vi "Kpro Read String Pot 2016.vi"(0 "Read String Pot":bool, 1 "Feet of\nStainless to be\nUsed (Count) in":i32, 2 "Corrected Array in":dbl[][](array[numeric]), 3 "Flow":dbl, 4 "Increment":bool, 5 "Finished In":bool, 6 "Depth Cluster in":T1, 7 "error in (no error)":errorcluster, 8 "String Pot \nSlope in":dbl=1.7339999675750732 format="%.2f", 9 "Sensor Cluster In in":T3, 10 "Descriptions":string[](array[string]), 11 "Zeroed Pressure in":dbl format="%.2f", 12 "Array in":refnum<k24>[](array[refnum]), 14 "Output KPRO in":path=path "c:/junk.dat") -> (18 "Sensor Cluster 2":T3, 19 "IK":dbl, 20 "Array out":refnum<k24>[](array[refnum]), 21 "Boolean":bool, 22 "Boolean 2":bool, 23 "Enum":T2(ring), 24 "Feet of\nStainless to be\nUsed (Count) out":i32, 25 "Depth Cluster out":T1, 26 "Corrected Array out":dbl[][](array[numeric]))   [LabVIEW 2016]
uses:
  Waterloo DAQ/controls/MCC DAQ Readings.ctl
  C:/Program Files (x86)/National Instruments/LabVIEW 2016/vi.lib/ULx/ULx_LV.dll
  Waterloo DAQ/controls/Kpro hydraulic measurement cluster.ctl
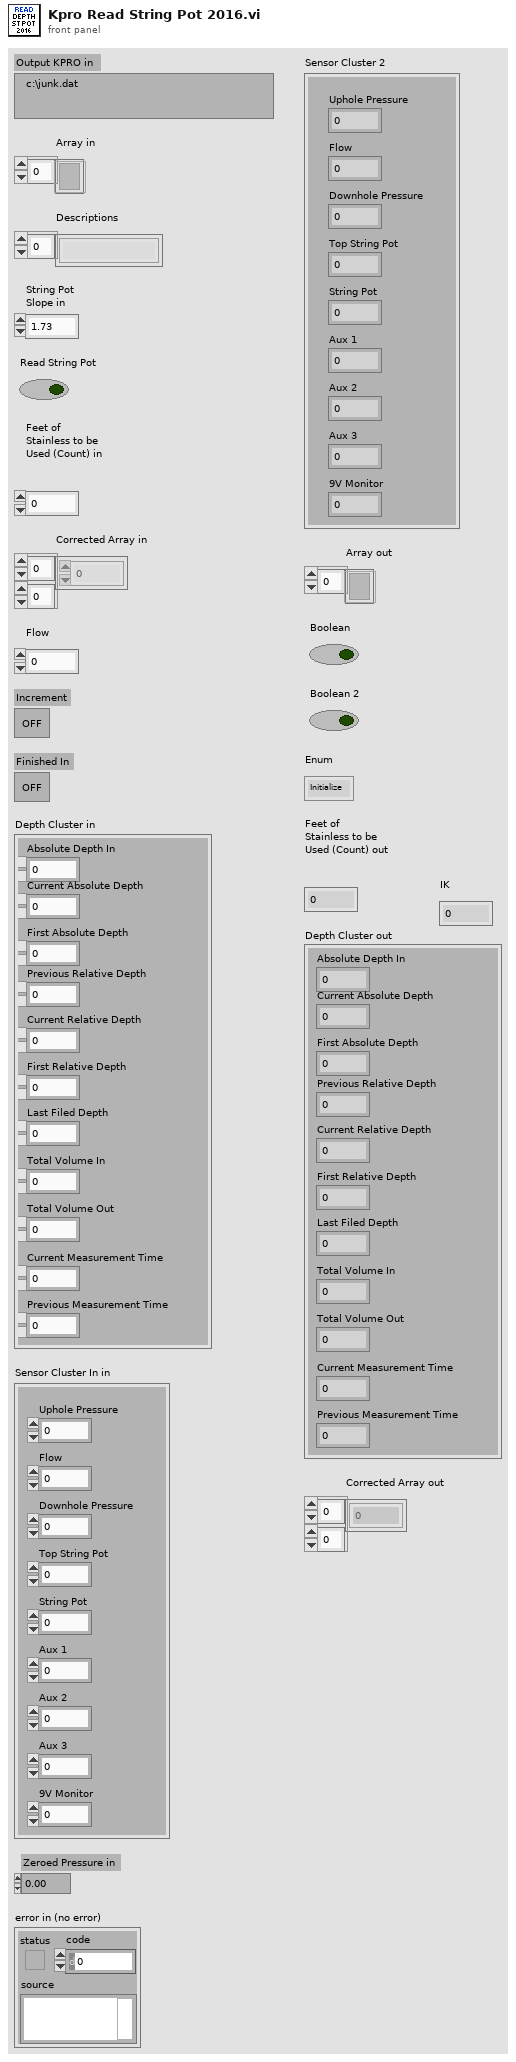
[diagram p1: front panel]
types:
  T1 = typedef "Kpro hydraulic measurement cluster.ctl" = cluster{"Absolute Depth In":dbl, "Current Absolute Depth":dbl, "First Absolute Depth":dbl, "Previous Relative Depth":dbl, "Current Relative Depth":dbl, "First Relative Depth":dbl, "Last Filed Depth":dbl, "Total Volume In":dbl, "Total Volume Out":dbl, "Current Measurement Time":dbl, "Previous Measurement Time":dbl}
  T2 = enum16{"Initialize", "Read", "Calc IK and generate Array", "Write Data & finish"}
  T3 = typedef "MCC DAQ Readings.ctl" = cluster{"Uphole Pressure":dbl, "Flow":dbl, "Downhole Pressure":dbl, "Top String Pot":dbl, "String Pot":dbl, "Aux 1":dbl, "Aux 2":dbl, "Aux 3":dbl, "9V Monitor":dbl}
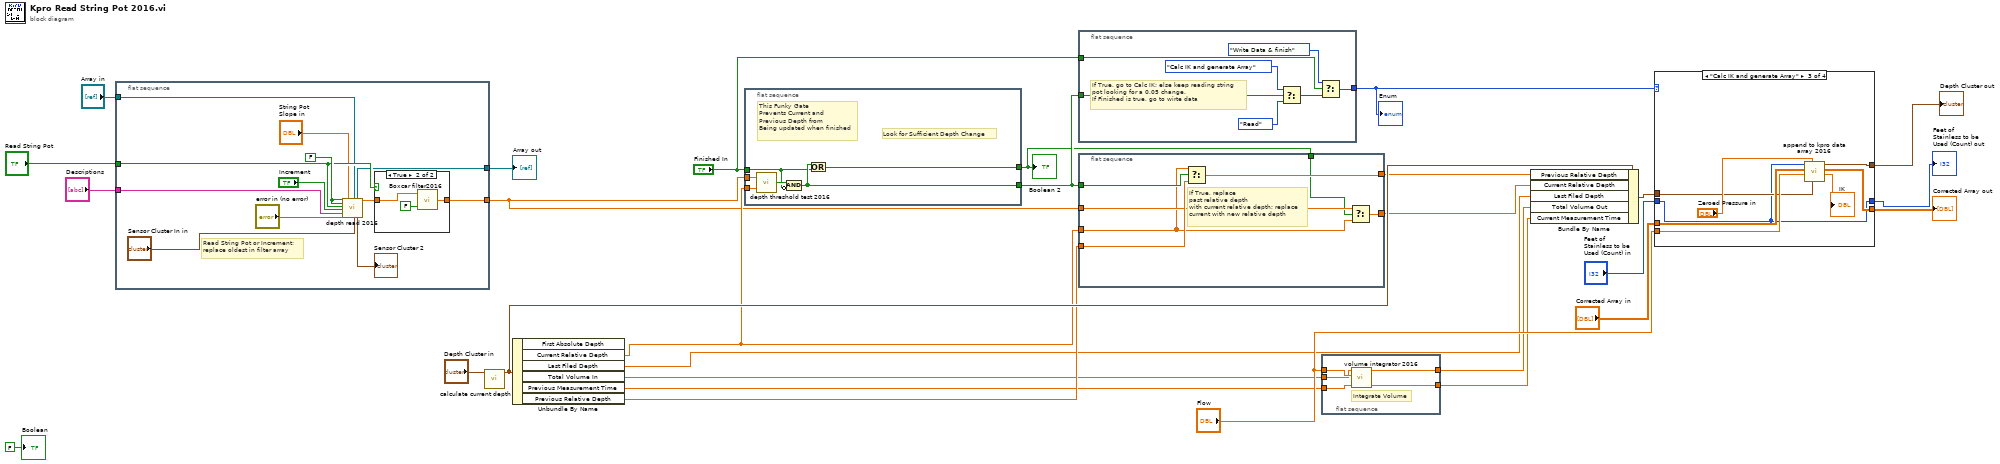
[diagram p0: block diagram]
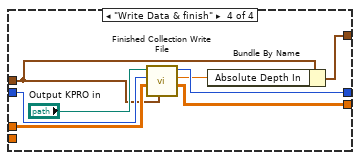
[diagram p4: hidden frame]
diagram:
  n1 = flat-sequence {
    tunnel: [w37] -> w5
    tunnel: "Read String Pot" -> [w36]
    tunnel: "Descriptions" -> [w35]
    tunnel: [w32] -> w27
    tunnel: "Array in" -> [w31]
    frame #0 {
      w39 = FALSE
      # "Read String Pot or Increment;\nreplace oldest in filter array"
      n2 = call "depth read 2016.vi"("Debug"=w39, "Initialize Debug"=w39, "Read String Pot"=w36, "Increment Button"="Increment", "Descriptions"=w35, "error in (no error)"="error in (no error)", "String Pot \nSlope"="String Pot \nSlope in", "Array in"=w31, "Sensor Cluster In"="Sensor Cluster In in") -> ("Array out"=w32:refnum<k24>[], "Sensor Cluster 2"=→"Sensor Cluster 2":T3, "Depth"=w40:dbl)  [unwired: 7 in, 1 out]
      n3 = case shown="True" w36 {
        tunnel: w40 -> [w41 w43]
        tunnel: [w41 w42] -> w37
        frame False {
        }
        frame True {
          n4 = call "Boxcar filter2016.vi"("Initialize"=FALSE, "Filter Input"=w43) -> ("Filter Output"=w42:dbl)  [unwired: 1 in]
        }
      }
    }
  }
  n5 = call "calculate current depth.vi"("Cluster in"="Depth Cluster in") -> ("Cluster out"=w17:T1)  [unwired: 10 in]
  n6 = Unbundle By Name(w17) -> ("Current Relative Depth"=w7:dbl, "Last Filed Depth"=w12:dbl, "Total Volume In"=w8:dbl, "Previous Measurement Time"=w14:dbl, "Previous Relative Depth"=w15:dbl)  [unwired: 1 out]
  n7 = flat-sequence {
    tunnel: [w49] -> w1
    tunnel: [w48] -> w2
    tunnel: "Finished In" -> [w47]
    tunnel: w5 -> [w46]
    tunnel: w7 -> [w45]
    frame #0 {
      # "Look for Sufficient Depth Change"
      # "This Funky Gate\nPrevents Current and \nPrevious Depth from \nBeing updated when finished"
      n8 = call "depth threshold test 2016.vi"("Depth\nPrevious"=w45, "Depth \nCurrent"=w46) -> ("Threshold\nExceeded"=w50:bool)
      n9 = Compound Arithmetic op=AND(w50, invert w47) -> (w48:bool)
      n10 = Or(x=w48, y=w47) -> (x .or. y?=w49:bool)
    }
  }
  n11 = flat-sequence {
    tunnel: [w57] -> w20
    tunnel: w2 -> [w55]
    tunnel: "Finished In" -> [w54]
    frame #0 {
      # "If True, go to Calc IK; else keep reading string pot looking for a 0.05 change.\nIf Finished is true, go to wirte data"
      n12 = Select(t=T2."Calc IK and generate Array", s=w55, f=T2."Read") -> (s? t:f=w56:T2)
      n13 = Select(t=T2."Write Data & finish", s=w54, f=w56) -> (s? t:f=w57:T2)
    }
  }
  n14 = flat-sequence {
    tunnel: [w64] -> w10
    tunnel: w15 -> [w63]
    tunnel: [w62] -> w11
    tunnel: w2 -> [w61]
    tunnel: w5 -> [w60]
    tunnel: w7 -> [w59]
    tunnel: w1 -> [w58]
    frame #0 {
      # "If True, replace\npast relative depth\nwith current relative depth; replace\ncurrent with new relative depth"
      n15 = Select(t=w59, s=w61, f=w63) -> (s? t:f=w64:dbl)
      n16 = Select(t=w60, s=w58, f=w59) -> (s? t:f=w62:dbl)
    }
  }
  n17 = flat-sequence {
    tunnel: w14 -> [w69]
    tunnel: [w68] -> w13
    tunnel: "Flow" -> [w67]
    tunnel: w8 -> [w66]
    tunnel: [w65] -> w9
    frame #0 {
      # "Integrate Volume"
      n18 = call "volume integrator 2016.vi"("Previous Time (sec)"=w69, "Flow"=w67, "Total Volume in"=w66) -> ("Current Time (sec)"=w68:dbl, "Total Volume Out"=w65:dbl)  [unwired: 3 in]
    }
  }
  n19 = Bundle By Name(cluster=w17, "Previous Relative Depth"=w10, "Current Relative Depth"=w11, "Last Filed Depth"=w12, "Total Volume Out"=w9, "Current Measurement Time"=w13) -> (w18:T1)
  n20 = case shown="\"Calc IK and generate Array\"" w20 {
    tunnel: "Corrected Array in" -> [w71 w75 w83 w89]
    tunnel: [w71 w75 w82 w87] -> w22
    tunnel: "Feet of\nStainless to be\nUsed (Count) in" -> [w70 w73 w77 w90]
    tunnel: "Flow" -> [_ _ w81 _]
    tunnel: [w72 w74 w80 w85] -> w19
    tunnel: w18 -> [w72 w74 w78 w86]
    tunnel: [w70 w73 w77 w88] -> w25
    frame "Initialize", Default {
    }
    frame "Read" {
    }
    frame "Calc IK and generate Array" {
      n21 = call "append to kpro data array 2016.vi"("Cluster in"=w78, "Zeroed Pressure"="Zeroed Pressure in", "Flow"=w81, "Corrected Array in"=w83, "Feet of\nStainless to be\nUsed (Count) in"=w77) -> ("IK"=→"IK":dbl, "Array"=w82:dbl[][], "Cluster out 2"=w80:T1)  [unwired: 4 in]
    }
    frame "Write Data & finish" {
      n22 = call "Finished Collection Write File.vi"("Cluster in"=w86, "Corrected Array in"=w89, "Feet of\nStainless to be\nUsed (Count) in"=w90, "Output KPRO"="Output KPRO in") -> ("Corrected Array out"=w87:dbl[][], "Depth to \nbe Used \n(Feet)"=w84:sgl, "Feet of\nStainless to be\nUsed (Count) out"=w88:i32)  [unwired: 5 in]
      n23 = Bundle By Name(cluster=w86, "Absolute Depth In"=w84) -> (w85:T1)
    }
  }
  "Feet of\nStainless to be\nUsed (Count) out" <- w25
  "Corrected Array out" <- w22
  "Depth Cluster out" <- w19
  "Array out" <- w27
  "Enum" <- w20
  "Boolean" <- FALSE
  "Boolean 2" <- w1
